vi "Work.vi"(2 "ThreadIdIn":u64, 3 "Dll Path":path) -> (0 "CPUThreadAffinity":u64, 1 "UsedThreadId":u64)   [LabVIEW 2013]
panel:
  out "Counter":i32
  out "error out":errorcluster
  in  "stop":bool
  in  "error in (no error)":errorcluster
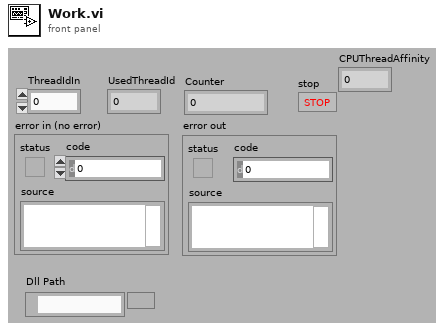
[diagram p1: front panel]
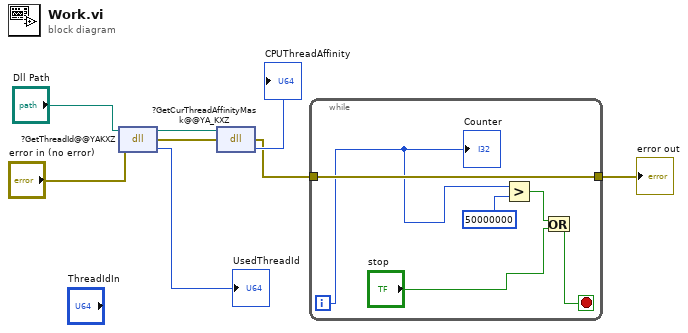
[diagram p0: block diagram]
diagram:
  n1 = dll-call lib="ThreadDll.dll" fn="?GetThreadId@@YAKXZ"(path in="Dll Path", error in="error in (no error)") -> (path out=w4:path, error out=w6:errorcluster, "return type"=→"UsedThreadId":u64)  [unwired: 1 in]
  n2 = dll-call lib="ThreadDll.dll" fn="?GetCurThreadAffinityMask@@YA_KXZ"(path in=w4, error in=w6) -> (error out=w1:errorcluster, "return type"=→"CPUThreadAffinity":u64)  [unwired: 1 in, 1 out]
  n3 = while {
    tunnel: w1 -> [w14]
    tunnel: [w14] -> w3
    i -> [w12]
    stop <- w9 stop-if-true
    n4 = Greater?(x=w12, y=50000000) -> (0:w11:bool)
    n5 = Or(x=w11, y="stop") -> (x .or. y?=w9:bool)
    "Counter" <- w12
  }
  "error out" <- w3
